vi "ACT_7_Task2_vikas.potluri.vi"() -> ()   [LabVIEW 2016]
panel:
  out "Numeric":dbl
  out "Loop Count":i32
  in  "Starting Value":i32
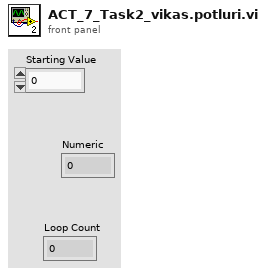
[diagram p1: front panel]
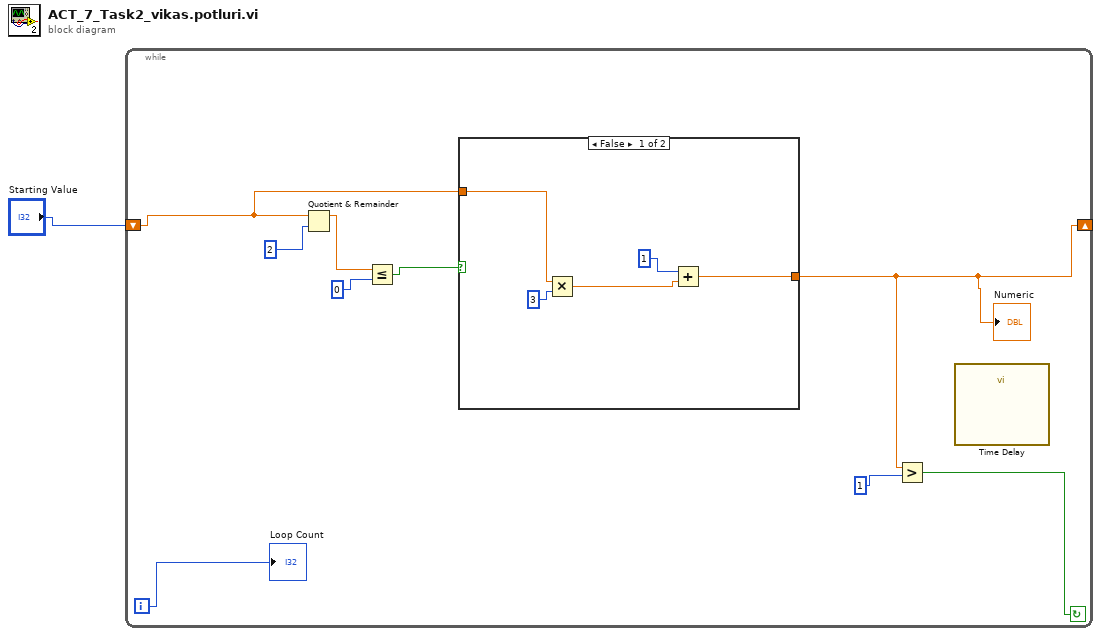
[diagram p0: block diagram]
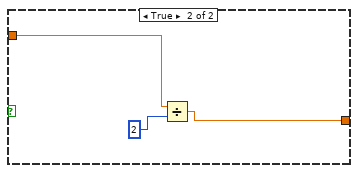
[diagram p2: hidden frame]
diagram:
  n1 = while {
    shift-right: [w2] -> _
    shift-left: "Starting Value" -> [w6]
    i -> [w10]
    stop <- w4 continue-if-true
    n2 = Quotient & Remainder(x=w6, y=2) -> (x-y*floor(x/y)=w8:dbl)  [unwired: 1 out]
    n3 = Less Or Equal?(x=w8, y=0) -> (x <= y?=w3:bool)
    n4 = case shown="False" w3 {
      tunnel: w6 -> [w15 w16]
      tunnel: [w11 w17] -> w2
      frame False {
        n5 = Multiply(x=w15, y=3) -> (x*y=w13:dbl)
        n6 = Add(x=1, y=w13) -> (x+y=w11:dbl)
      }
      frame True {
        n7 = Divide(x=w16, y=2) -> (x/y=w17:dbl)
      }
    }
    "Numeric" <- w2
    n8 = Greater?(x=w2, y=1) -> (0:w4:bool)
    n9 = call "Time Delay"() -> ()  [unwired: 11 in, 1 out]
    "Loop Count" <- w10
  }
